vi "Periodic Tasks.vi"(11 "navX Device":T2={"Interface"={"Protocol"=enum."SERIAL", "Update Rate (4Hz-60Hz)"=4, "navX Open TypeDef"=variant}, "Notify Packet"=refnum, "Loop VI Refnum"=refnum, "Ready to Close Occurrence Refnum"=refnum} {"Interface"."Update Rate (4Hz-60Hz)" min=4 max=60 step=1}) -> ()   [LabVIEW 2015]
doc: "This VI runs in parallel to other tasks. It can contain as many user-defined periodic loops as you need. These can carry out PID or other sorts of timed response."
uses:
  navx-mxp/labview/navX Library v2/TypeDefs/Z900_navX_DeviceTypeDef.ctl
  navx-mxp/labview/navX Library v2/TypeDefs/Z900_navX_ProtocolTypeDef.ctl
  navx-mxp/labview/navX Library v2/TypeDefs/Z900_navX_NotifyPacketTypeDef.ctl
  navx-mxp/labview/navX Library v2/TypeDefs/Z900_navX_ActionTypeDef.ctl
  <vilib>/Rock Robotics/WPI/Utilities/WPI_GetSetVariantRefNum.vi
  Robot Global Data.vi
  navx-mxp/labview/navX Library v2/navX Library v2.lvlib
panel:
  in  "PID gains":T1={"proportional gain (Kc)"=0.005, "integral time (Ti, min)"=3e-06, "derivative time (Td, min)"=0.0} {"derivative time (Td, min)" format="%.16f"; "integral time (Ti, min)" format="%.16f"; "proportional gain (Kc)" format="%.16f"}
  out "Angle Out":dbl
  out "Waveform Chart":dbl(graph)
  out "Internal error out 2":errorcluster
  out "YAW 2":dbl
  out "Roll 2":dbl
  out "Pitch 2":dbl
  out "Heading 2":dbl
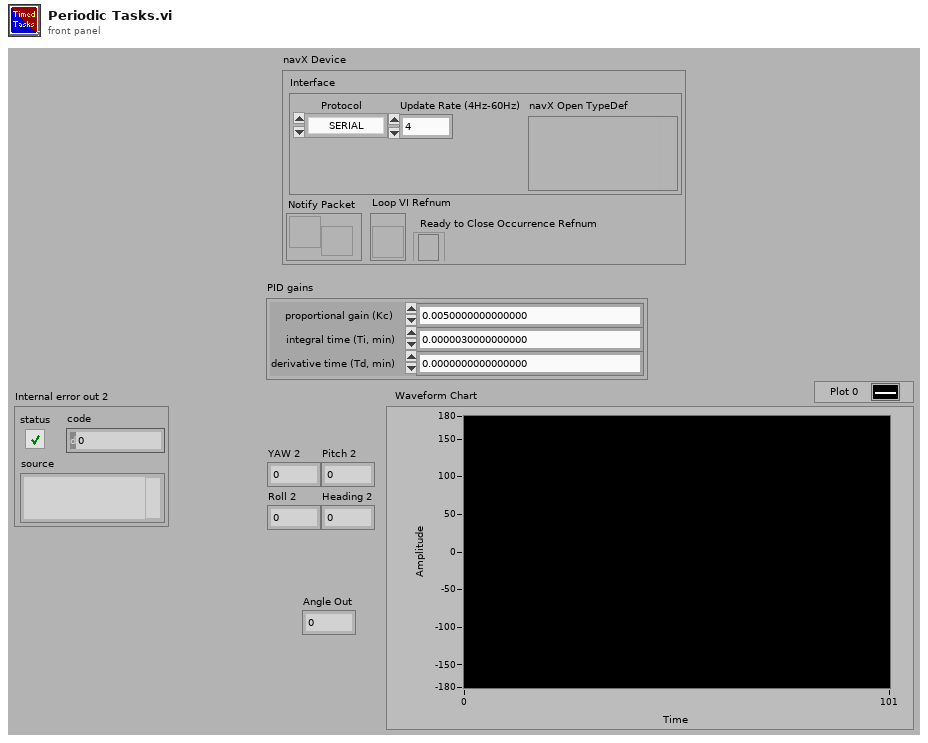
[diagram p1: front panel]
types:
  T1 = cluster{"proportional gain (Kc)":dbl, "integral time (Ti, min)":dbl, "derivative time (Td, min)":dbl}
  T2 = typedef "navX Library v2.lvlib/Z900_navX_DeviceTypeDef.ctl" = cluster{"Interface":cluster{"Protocol":T3, "Update Rate (4Hz-60Hz)":u8, "navX Open TypeDef":variant}, "Notify Packet":refnum<notifier>, "Loop VI Refnum":refnum<vi>, "Ready to Close Occurrence Refnum":refnum<k4>}
  T3 = typedef "navX Library v2.lvlib/Z900_navX_ProtocolTypeDef.ctl" = enum16{"SERIAL", "I2C", "SPI"}
  T4 = typedef "WPI_JoystickDevRef.ctl" = cluster{"Device":T5}
  T5 = typedef "WPI_JoystickDeviceEnum.ctl" = enum16{"USB 0", "USB 1", "USB 2", "USB 3", "USB 4", "USB 5"}
  T6 = cluster{"Axes[0]":dbl, "Axes[1]":dbl, "Axes[2]":dbl, "Axes[3]":dbl, "Axes[4]":dbl, "Axes[5]":dbl, "Axes[6]":dbl, "Axes[7]":dbl, "Axes[8]":dbl}
  T7 = cluster{"Buttons[0]":bool, "Buttons[1]":bool, "Buttons[2]":bool, "Buttons[3]":bool, "Buttons[4]":bool, "Buttons[5]":bool, "Buttons[6]":bool, "Buttons[7]":bool, "Buttons[8]":bool}
  T8 = cluster{"Yaw":dbl, "Roll":dbl, "Pitch":dbl, "Heading":dbl, "Fused Heading":dbl}
  T9 = typedef "WPI_MotorControlDeviceRef.ctl" = cluster{"DeviceStatus":errorcluster, "Type":T10, "PWM":cluster{"PWM Channel":T11, "DeadBand":T12}, "CAN":cluster{"Device Number":u8, "Control Mode":T13, "Semaphore":T14, "Max Vout":dbl, "TalonSRX Control Mode":T15}, "Invert":bool}
  T10 = typedef "WPI_MotorControlType.ctl" = enum16{"PWM", "CAN", "CANTalonSRX"}
  T11 = typedef "FPGA_DIOPWMChannel.ctl" = enum8{"PWM 0", "PWM 1", "PWM 2", "PWM 3", "PWM 4", "PWM 5", "PWM 6", "PWM 7", "PWM 8", "PWM 9", "PWM MXP 0", "PWM MXP 1", "PWM MXP 2", "PWM MXP 3", "PWM MXP 4", "PWM MXP 5", "PWM MXP 6", "PWM MXP 7", "PWM MXP 8", "PWM MXP 9", "Invalid"}
  T12 = typedef "WPI_PWMDeadband.ctl" = cluster{"Name":string, "maxPositivePwm":i32, "minPositivePwm":i32, "centerPwm":i32, "maxNegativePwm":i32, "minNegativePwm":i32, "angularRange":u16}
  T13 = typedef "WPI_CANJaguar_ControlMode.ctl" = enum8{"Percent VBus", "Current", "Speed", "Position", "Voltage"}
  T14 = typedef "Semaphore RefNum" = refnum<k1>
  T15 = typedef "WPI_CANTalonSRX_APIControlMode.ctl" = enum8{"Percent VBus", "Speed", "Position", "Slave", "Unchanged / Invalid", "Voltage Compensation", "Current", "Motion Profile"}
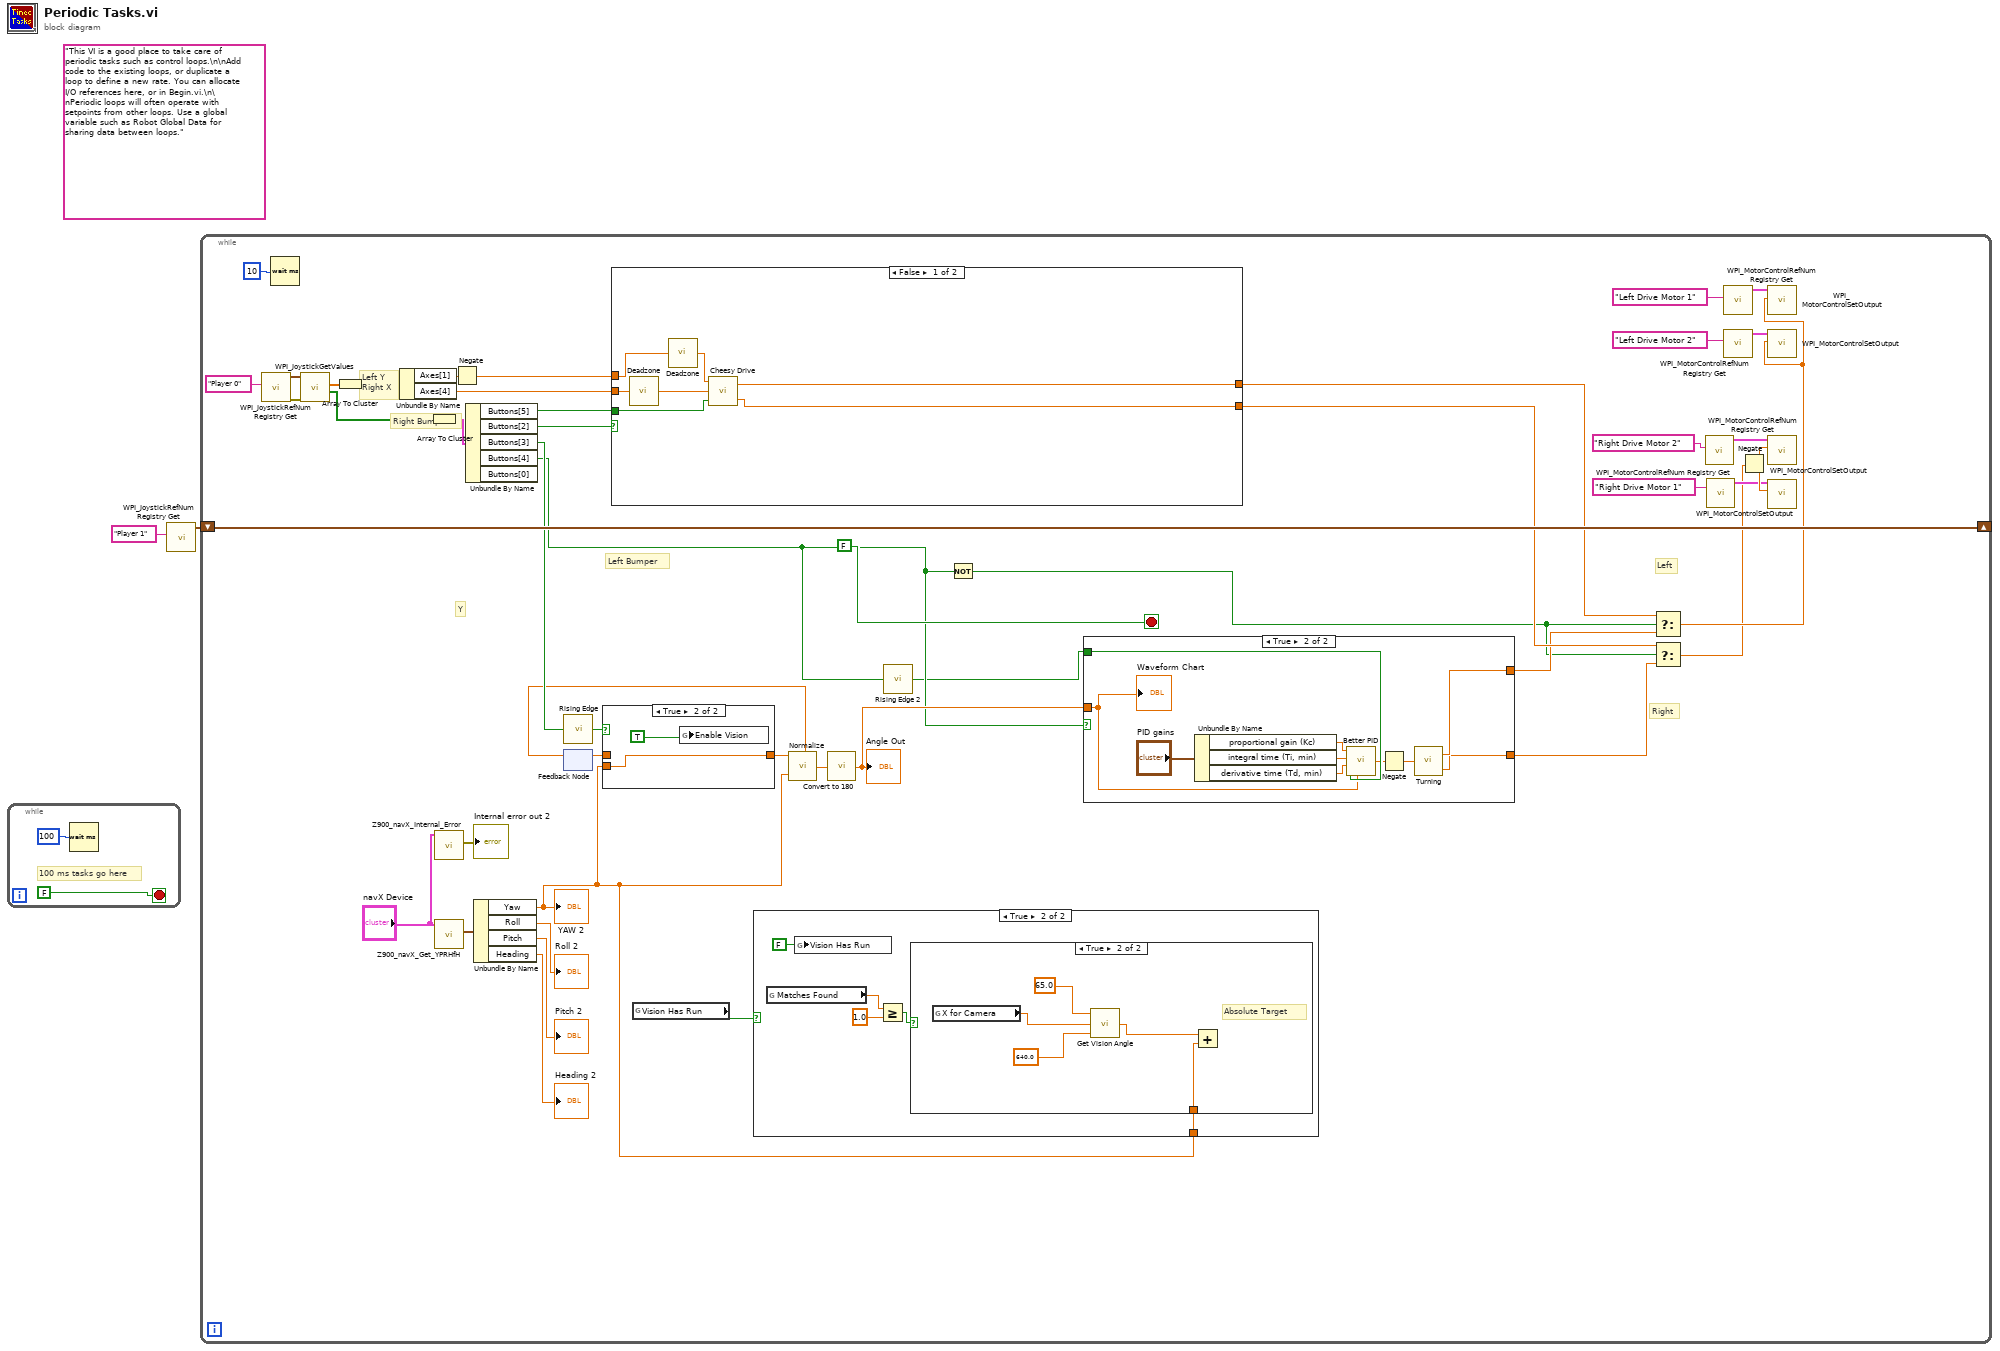
[diagram p0: block diagram]
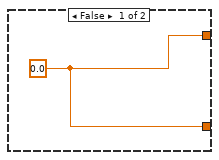
[diagram p4: hidden frame]
diagram:
  (unwired) "This VI is a good place to take care of periodic tasks such as control loops.\n\nAdd code to the existing loops, or duplicate a loop to define a new rate. You can allocate I/O references here, or in Begin.vi.\n\nPeriodic loops will often operate with setpoints from other loops. Use a global variable such as Robot Global Data for sharing data between loops."
  n1 = while {
    stop <- FALSE stop-if-true
    # "100 ms tasks go here"
    n2 = Wait (ms)(milliseconds to wait=u32 100) -> ()  [unwired: 1 out]
  }
  n3 = call <vilib>:"WPI_JoystickRefNum Registry Get.vi"("refnum name"="Player 1") -> ("JoystickDevRef"=w1:T4)  [unwired: 9 in, 1 out]
  n4 = while {
    shift-right: [w50] -> _
    shift-left: w1 -> [w50]
    stop <- FALSE stop-if-true
    # "Y"
    # "Left Bumper"
    # "Right"
    # "Left"
    # "Right Bumper"
    # "Left Y\nRight X"
    n5 = call <vilib>:"WPI_JoystickRefNum Registry Get.vi"("refnum name"="Player 0") -> ("error out"=w36:errorcluster, "JoystickDevRef"=w37:T4)  [unwired: 1 in, 8 out]
    n6 = Wait (ms)(milliseconds to wait=u32 10) -> ()  [unwired: 1 out]
    n7 = call <vilib>:"WPI_JoystickGetValues.vi"("error in (no error)"=w36, "JoystickDevRef"=w37) -> ("Buttons"=w47:bool[], "Axes"=w49:dbl[])  [unwired: 5 in, 3 out]
    n8 = Array To Cluster(array=w49) -> (cluster=w48:T6)
    n9 = Unbundle By Name(w48) -> ("Axes[1]"=w40:dbl, "Axes[4]"=w43:dbl)
    n10 = Array To Cluster(array=w47) -> (cluster=w46:T7)
    n11 = call "Z900_navX_Internal_Error.vi"("navX Device"="navX Device") -> ("Internal error out"=→"Internal error out 2":errorcluster)  [unwired: 8 in, 2 out]
    n12 = call "Z900_navX_Get_YPRHfH.vi"("navX Device"="navX Device") -> ("YRPHfH"=w23:T8)  [unwired: 7 in, 3 out]
    n13 = Negate(x=w40) -> (-x=w39:dbl)
    n14 = Unbundle By Name(w46) -> ("Buttons[5]"=w44:bool, "Buttons[2]"=w45:bool, "Buttons[3]"=w27:bool, "Buttons[4]"=w8:bool)  [unwired: 1 out]
    n15 = Unbundle By Name(w23) -> ("Yaw"=w5:dbl, "Roll"=→"Roll 2":dbl, "Pitch"=→"Pitch 2":dbl, "Heading"=→"Heading 2":dbl)
    "YAW 2" <- w5
    n16 = call "Rising Edge.vi"("Button Pressed?"=w27) -> ("Bool Output"=w9:bool)
    n17 = feedback #1() -> (w20:dbl)  [unwired: 1 in]
    n18 = case shown="True" w9 {
      tunnel: [w73 w75] -> w17
      tunnel: w5 -> [_ w75]
      tunnel: w20 -> [w73 _]
      frame False {
      }
      frame True {
        n19 = global write "Robot Global Data.vi" "Enable Vision"(TRUE) -> ()
      }
    }
    n20 = feedback-in #1(w17) -> ()
    n21 = case shown="False" w45 {
      tunnel: w44 -> [w80 _]
      tunnel: w39 -> [w76 w84]
      tunnel: w43 -> [w79 w83]
      tunnel: [w78 w84] -> w16
      tunnel: [w77 w83] -> w15
      frame False {
        n22 = call "Deadzone.vi"("Input"=w79) -> ("Output"=w81:dbl)
        n23 = call "Deadzone.vi"("Input"=w76) -> ("Output"=w82:dbl)
        n24 = call "Cheesy Drive.vi"("Quick Turn"=w80, "Turn"=w81, "Throttle"=w82) -> ("Right Motor"=w77:dbl, "Left Motor"=w78:dbl)
      }
      frame True {
        # "gyr"
      }
    }
    n25 = global read "Robot Global Data.vi" "Vision Has Run"() -> (w6:bool)
    n26 = case shown="True" w6 {
      tunnel: w5 -> [_ w52]
      frame False {
      }
      frame True {
        n27 = global read "Robot Global Data.vi" "Matches Found"() -> (w54:dbl)
        n28 = global write "Robot Global Data.vi" "Vision Has Run"(FALSE ("Vision Has Run")) -> ()
        n29 = Greater Or Equal?(x=w54, y=1.0) -> (x >= y?=w55:bool)
        n30 = case shown="True" w55 {
          tunnel: w52 -> [_ w57]
          frame False {
          }
          frame True {
            # "Absolute Target"
            n31 = global read "Robot Global Data.vi" "X for Camera"() -> (w59:dbl)
            n32 = call "Get Vision Angle.vi"("Camera Resolution (in pixels, along the axis you want)"=640.0, "Object Position (in pixels)"=w59, "Camer FOV (in degrees)"=65.0) -> ("Object Position (in degrees)"=w58:dbl)
            n33 = Add(x=w58, y=w57) -> ()  [unwired: 1 out]
          }
        }
      }
    }
    n34 = call "Normalize.vi"("Current Angle"=w5, "Initial Angle"=w17) -> ("Normalized Angle"=w19:dbl)
    n35 = call "Convert to 180.vi"("Angle In"=w19) -> ("Angle Out"=w18:dbl)
    "Angle Out" <- w18
    n36 = call "Rising Edge 2.vi"("Button Pressed?"=w8) -> ("Bool Output"=w7:bool)
    n37 = Not(x=w8) -> (.not. x?=w10:bool)
    n38 = case shown="True" w8 {
      tunnel: w18 -> [_ w69]
      tunnel: [w62 w72] -> w12
      tunnel: [w62 w71] -> w11
      tunnel: w7 -> [_ w70]
      frame False {
        w62 = 0.0 ("Left Motor")
      }
      frame True {
        n39 = Unbundle By Name("PID gains") -> ("proportional gain (Kc)"=w65:dbl, "integral time (Ti, min)"=w64:dbl, "derivative time (Td, min)"=w63:dbl)
        n40 = call "Better PID.vi"("Process Variable"=w69, "Reset Error Accumulater"=w70, "D"=w63, "I"=w64, "P"=w65) -> ("Out"=w68:dbl)  [unwired: 1 in]
        n41 = Negate(x=w68) -> (-x=w67:dbl)
        n42 = call "Turning.vi"("Turn Rate"=w67) -> ("Left Motor"=w72:dbl, "Right Motor"=w71:dbl)
        "Waveform Chart" <- w69
      }
    }
    n43 = Select(t=w16, s=w10, f=w12) -> (s? t:f=w14:dbl)
    n44 = Select(t=w15, s=w10, f=w11) -> (s? t:f=w13:dbl)
    n45 = call <vilib>:"WPI_MotorControlRefNum Registry Get.vi"("refnum name"="Right Drive Motor 2") -> ("MotorControlDevRef"=w29:T9)  [unwired: 9 in, 1 out]
    n46 = call <vilib>:"WPI_MotorControlRefNum Registry Get.vi"("refnum name"="Right Drive Motor 1") -> ("MotorControlDevRef"=w28:T9)  [unwired: 9 in, 1 out]
    n47 = call <vilib>:"WPI_MotorControlRefNum Registry Get.vi"("refnum name"="Left Drive Motor 1") -> ("MotorControlDevRef"=w33:T9)  [unwired: 9 in, 1 out]
    n48 = call <vilib>:"WPI_MotorControlRefNum Registry Get.vi"("refnum name"="Left Drive Motor 2") -> ("MotorControlDevRef"=w32:T9)  [unwired: 9 in, 1 out]
    n49 = Negate(x=w13) -> (-x=w41:dbl)
    n50 = call <vilib>:"WPI_MotorControlSetOutput.vi"("Output"=w14, "MotorControlDevRef"=w33) -> ()  [unwired: 7 in, 3 out]
    n51 = call <vilib>:"WPI_MotorControlSetOutput.vi"("Output"=w14, "MotorControlDevRef"=w32) -> ()  [unwired: 7 in, 3 out]
    n52 = call <vilib>:"WPI_MotorControlSetOutput.vi"("Output"=w41, "MotorControlDevRef"=w29) -> ()  [unwired: 7 in, 3 out]
    n53 = call <vilib>:"WPI_MotorControlSetOutput.vi"("Output"=w41, "MotorControlDevRef"=w28) -> ()  [unwired: 7 in, 3 out]
  }
